vi "NanonisProperties_raw.vi"(0 "Application ref in":refnum<vi>, 5 "Position (nm)":cluster{"X":dbl, "Z":dbl, "Y":dbl}, 11 "error in (no error)":errorcluster, 12 "Z Write?":bool) -> (4 "Application ref out":refnum<vi>, 8 "Current (pA)":sgl format="%#_6p", 10 "Z Read (m)":sgl format="%#_6p", 15 "error out":errorcluster)   [LabVIEW 2019]
uses:
  <userlib>/Nanonis Prog Interface V5/Nanonis Prog Interface.lvlib
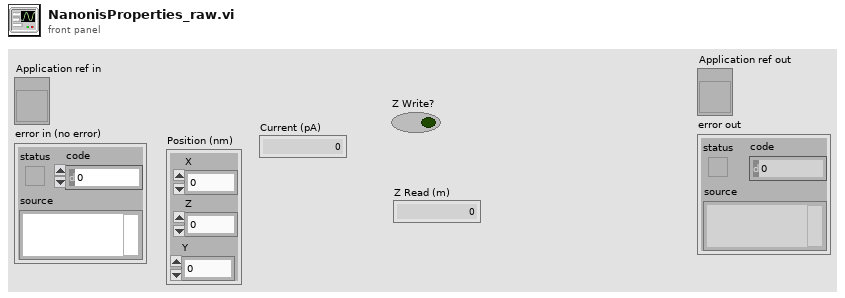
[diagram p1: front panel]
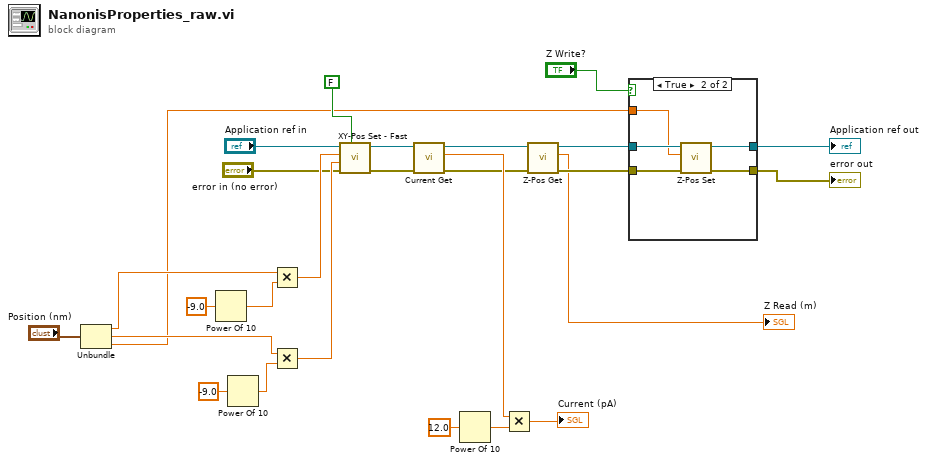
[diagram p0: block diagram]
diagram:
  n1 = Unbundle("Position (nm)") -> ("X"=w3:dbl, "Z"=w2:dbl, "Y"=w1:dbl)
  n2 = Power Of 10(x=-9.0) -> (10^x=w26:dbl)
  n3 = Power Of 10(x=-9.0) -> (10^x=w24:dbl)
  n4 = Multiply(x=w3, y=w26) -> (x*y=w22:dbl)
  n5 = Multiply(x=w2, y=w24) -> (x*y=w21:dbl)
  n6 = call <userlib>:"XY-Pos Set - Fast.vi"("Wait end-of-motion (T=True)"=FALSE, "error in (no error)"="error in (no error)", "Y (m)"=w21, "X (m)"=w22, "Application ref in"="Application ref in") -> ("error out"=w7:errorcluster, "Application ref out"=w8:refnum<vi>)  [unwired: 4 in]
  n7 = call <userlib>:"Current Get.vi"("Error in (no error)"=w7, "Application ref in"=w8) -> ("Error out"=w15:errorcluster, "Current (A)"=w17:sgl, "Application ref out"=w16:refnum<vi>)  [unwired: 5 in]
  n8 = Power Of 10(x=12.0) -> (10^x=w18:dbl)
  n9 = Multiply(x=w17, y=w18) -> (x*y=→"Current (pA)":dbl)
  n10 = call <userlib>:"Z-Pos Get.vi"("error in (no error)"=w15, "Application ref in"=w16) -> ("error out"=w13:errorcluster, "Z position (m)"=→"Z Read (m)":sgl, "Application ref out"=w14:refnum<vi>)  [unwired: 7 in]
  n11 = case shown="True" "Z Write?" {
    tunnel: w14 -> [w29 w34]
    tunnel: w13 -> [w28 w33]
    tunnel: [w29 w32] -> w12
    tunnel: [w28 w31] -> w11
    tunnel: w1 -> [_ w30]
    frame False {
    }
    frame True {
      n12 = call <userlib>:"Z-Pos Set.vi"("error in (no error)"=w33, "Z position (m)"=w30, "Application ref in"=w34) -> ("error out"=w31:errorcluster, "Application ref out"=w32:refnum<vi>)  [unwired: 7 in]
    }
  }
  "Application ref out" <- w12
  "error out" <- w11
